vi "LEP_RV_WriteFlagsToXML.vi"(8 "error in":errorcluster, 9 "Linker flags":string, 10 "Compiler flags":string, 11 "XML file refnum":refnum<file>) -> (0 "error out":errorcluster, 3 "XML file refnum":refnum<file>)   [LabVIEW 2011]
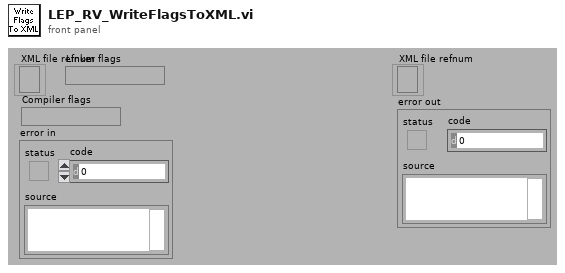
[diagram p1: front panel]
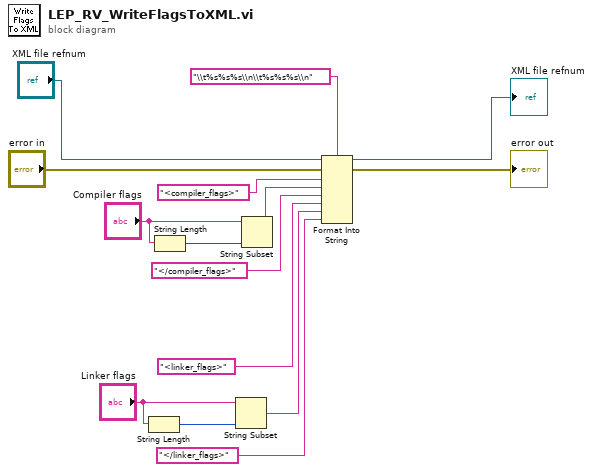
[diagram p0: block diagram]
diagram:
  n1 = String Length(string="Linker flags") -> (length=w1:i32)
  n2 = String Length(string="Compiler flags") -> (length=w2:i32)
  n3 = String Subset(string="Linker flags", length (rest)=w1) -> (substring=w6:string)  [unwired: 1 in]
  n4 = String Subset(string="Compiler flags", length (rest)=w2) -> (substring=w8:string)  [unwired: 1 in]
  n5 = Format Into String(format string="\\t%s%s%s\\n\\t%s%s%s\\n", initial string="XML file refnum", error in="error in", "<compiler_flags>" ("input 1"), w8, "</compiler_flags>" ("input 2"), "<linker_flags>" ("input 1"), w6, "</linker_flags>" ("input 2")) -> (resulting string=→"XML file refnum":refnum<file>, error out=→"error out":errorcluster)
